vi "Instrument Retrieve Record.vi"(8 "error in (no error)":errorcluster, 11 "Statement Refnum":T2) -> (0 "error out":errorcluster, 2 "Instrument":T1, 3 "Statement Refnum":T2)   [LabVIEW 2011]
uses:
  SI.LIB/ODBC/SQL Controls/Statement Refnum.ctl
  Instrument Record.ctl
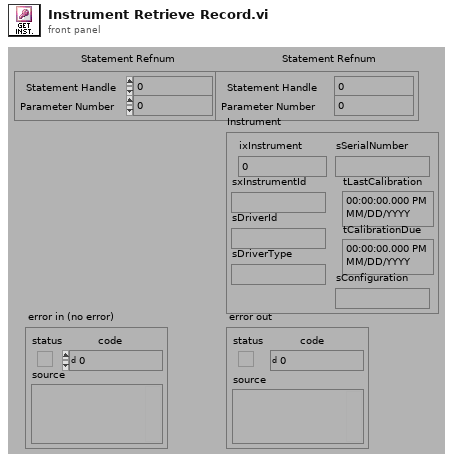
[diagram p1: front panel]
types:
  T1 = typedef "Instrument Record.ctl" = cluster{"ixInstrument":i32, "sxInstrumentId":string, "sDriverId":string, "sDriverType":string, "sSerialNumber":string, "tLastCalibration":timestamp, "tCalibrationDue":timestamp, "sConfiguration":string}
  T2 = typedef "Statement Refnum.ctl" = cluster{"Statement Handle":i32, "Parameter Number":u16}
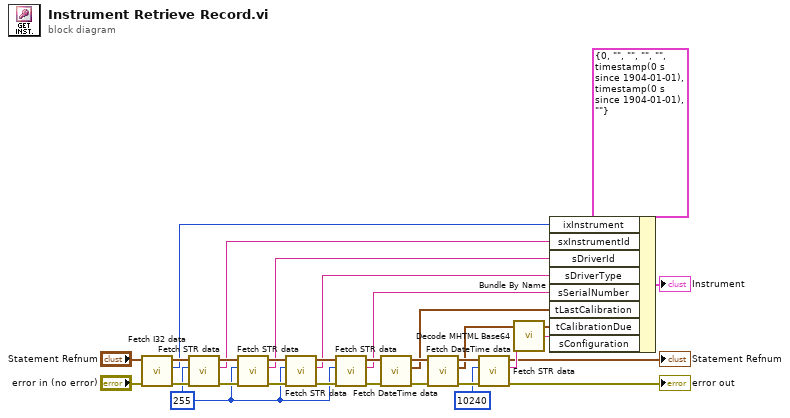
[diagram p0: block diagram]
diagram:
  w16 = 255 ("Buffer Size")
  n1 = call "Fetch I32 data.vi"("error in (no error)"="error in (no error)", "Statement Refnum"="Statement Refnum") -> ("error out"=w28:errorcluster, "Data"=w7:i32, "Statement Refnum"=w27:T2)  [unwired: 3 out]
  n2 = call "Fetch STR data.vi"("error in (no error)"=w28, "Buffer Size"=w16, "Statement Refnum"=w27) -> ("error out"=w30:errorcluster, "Data"=w18:string, "Statement Refnum"=w29:T2)  [unwired: 2 out]
  n3 = call "Fetch STR data.vi"("error in (no error)"=w30, "Buffer Size"=w16, "Statement Refnum"=w29) -> ("error out"=w26:errorcluster, "Data"=w15:string, "Statement Refnum"=w25:T2)  [unwired: 2 out]
  n4 = call "Fetch STR data.vi"("error in (no error)"=w26, "Buffer Size"=w16, "Statement Refnum"=w25) -> ("error out"=w22:errorcluster, "Data"=w12:string, "Statement Refnum"=w19:T2)  [unwired: 2 out]
  n5 = call "Fetch STR data.vi"("error in (no error)"=w22, "Buffer Size"=w16, "Statement Refnum"=w19) -> ("error out"=w21:errorcluster, "Data"=w17:string, "Statement Refnum"=w20:T2)  [unwired: 2 out]
  n6 = call "Fetch DateTime data.vi"("error in (no error)"=w21, "Statement Refnum"=w20) -> ("error out"=w24:errorcluster, "Data"=w2:timestamp, "Statement Refnum"=w23:T2)  [unwired: 3 out]
  n7 = call "Fetch DateTime data.vi"("error in (no error)"=w24, "Statement Refnum"=w23) -> ("error out"=w10:errorcluster, "Data"=w1:timestamp, "Statement Refnum"=w11:T2)  [unwired: 3 out]
  n8 = call "Fetch STR data.vi"("error in (no error)"=w10, "Buffer Size"=10240, "Statement Refnum"=w11) -> ("error out"=→"error out":errorcluster, "Data"=w6:string, "Statement Refnum"=→"Statement Refnum":T2)  [unwired: 2 out]
  n9 = call "Decode MHTML Base64.vi"("Encoded String\n(Base64)"=w6) -> ("Decoded Binary\nString"=w5:string)  [unwired: 14 out]
  n10 = Bundle By Name(cluster=T1 {"ixInstrument"=0, "sxInstrumentId"="", "sDriverId"="", "sDriverType"="", "sSerialNumber"="", "tLastCalibration"=timestamp(0 s since 1904-01-01), "tCalibrationDue"=timestamp(0 s since 1904-01-01), "sConfiguration"=""} ("Station Information"), "ixInstrument"=w7, "sxInstrumentId"=w18, "sDriverId"=w15, "sDriverType"=w12, "sSerialNumber"=w17, "tLastCalibration"=w2, "tCalibrationDue"=w1, "sConfiguration"=w5) -> (→"Instrument":T1)
